vi "LVProjectShortcut_Global_Init.vi"(8 "error in":errorcluster, 11 "Object":T1) -> (0 "error out":errorcluster)   [LabVIEW 2017]
uses:
  <resource>/Framework/Providers/API/ItemRef.ctl
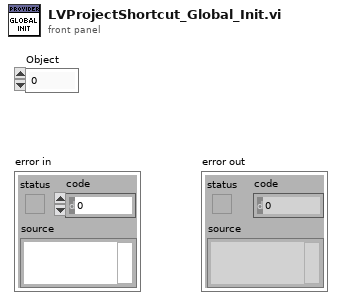
[diagram p1: front panel]
types:
  T1 = typedef "ItemRef.ctl" = u64
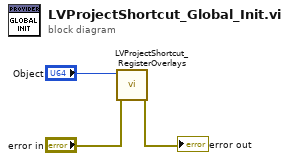
[diagram p0: block diagram]
diagram:
  n1 = call <resource>:"LVProjectShortcut_RegisterOverlays.vi"("error in"="error in", "Item"="Object") -> ("error out"=→"error out":errorcluster)  [unwired: 9 in]
